vi "WaveformGen.vi"(7 "Name (\"\" to Use UUID)":string="WaveformGen") -> ()   [LabVIEW 2020, in "CSM-SimWaveform.lvlib"]
doc: "------------- lvcsm -------------\n[CSMStates]\nItem 0 = \"Event Structure\"\nItem 1 = \"Idle\"\nItem 2 = \"CSM Documentation\"\nItem 3 = \"VI Reference\"\nItem 4 = \"Error Handler\"\nItem 5 = \"Critical Error\"\nItem 6 = \"Target Timeout Error\"\nItem 7 = \"Target Error\"\nItem 8 = \"Async Response\"\nItem 9 = \"Response\"\nItem 10 = \"Async Message Posted\"\nItem 11 = \"Initialize Core Data\"\nItem 12 = \"Exit\"\nItem 13 = \"Data: Initialize\"\nItem 14 = \"Data: Cleanup\"\nItem 15 = \"Events: Register\"\nItem 16 = \"Events: Unregister\"\nItem 17 = \"UI: Initialize\"\nItem 18 = \"UI: Cursor Set\"\nItem 19 = \"UI: Front Panel State\"\nItem 20 = \"Macro: Initialize\"\nItem 21 = \"Macro: Exit\"\nItem 22 = \"API: Configure\"\nItem 23 = \"API: Start\"\nItem 24 = \"API: Stop\"\nItem 25 = \"Action: GenerateWaveforms\"\n\n[CSMStatus]\nItem 0 = \"Acquired Waveform@\"\nItem 1 = \"Error Occurred@Error Handler\""
uses:
  _support/WfGenConf--Cluster.ctl
  d2f34d03-87f3-4da2-90aa-e537ed74afc7.vi
  29d10371-2bcf-4fcf-9d9e-e563f382a514.vi
  <userlib>/_NEVSTOP/Communicable State Machine(CSM)/AdvanceAPI/CSM - Revert Arguments-Safe String.vi
  <userlib>/_NEVSTOP/Communicable State Machine(CSM)/_Shared/Trim Single-line Text.vi
  <userlib>/_NEVSTOP/Communicable State Machine(CSM)/AdvanceAPI/CSM - Make String Arguments Safe.vi
  <userlib>/_NEVSTOP/Communicable State Machine(CSM)/AdvanceAPI/CSM - Break Down Multiple States String.vi
  <userlib>/_NEVSTOP/Communicable State Machine(CSM)/AdvanceAPI/CSM - Compact Multiple States.vi
  <userlib>/_NEVSTOP/Communicable State Machine(CSM)/AdvanceAPI/CSM - Keywords.vi
  <userlib>/_NEVSTOP/Communicable State Machine(CSM)/AdvanceAPI/CSM - List Modules.vi
  <userlib>/_NEVSTOP/Communicable State Machine(CSM)/Utility/CSM Data Type String.vi
  <userlib>/_NEVSTOP/Communicable State Machine(CSM)/addons/MassData-Parameter/_support/FGV-MassData(lvlibp).vi
  <userlib>/_NEVSTOP/Communicable State Machine(CSM)/addons/API-String-Arugments-Support/_Support/Convert API String Arguments to Data(variant).vi
  CSM-SimWaveform.lvlib
  <userlib>/_NEVSTOP/Communicable State Machine(CSM)/Communicable State Machine.lvlib
panel:
  in  "System Stop Button":bool
  in  "System Start Button":bool
  out "Running?":bool
  in  "Generate Rate":u32(knob)=17 scale=1.0..50.0
  out "diff(ms)":u32
  in  "WaveformGen Settings":T1(array[cluster])=[{"sampling info"={"Fs"=1000.0, "#s"=1000.0}, "phase"=0.0, "amplitude"=1.0, "frequency"=10.0, "range"=1.0, "Type"=enum."Sine", "Waveform Name"="Waveform 0"}, {"sampling info"={"Fs"=1000.0, "#s"=1000.0}, "phase"=0.0, "amplitude"=1.0, "frequency"=10.0, "range"=1.0, "Type"=enum."Triangle", "Waveform Name"="Waveform 1"}, {"sampling info"={"Fs"=1000.0, "#s"=1000.0}, "phase"=0.0, "amplitude"=1.0, "frequency"=10.0, "range"=1.0, "Type"=enum."Sawtooth", "Waveform Name"="Waveform 2"}, {"sampling info"={"Fs"=1000.0, "#s"=1000.0}, "phase"=0.0, "amplitude"=1.0, "frequency"=10.0, "range"=1.0, "Type"=enum."Square", "Waveform Name"="Waveform 3"}]
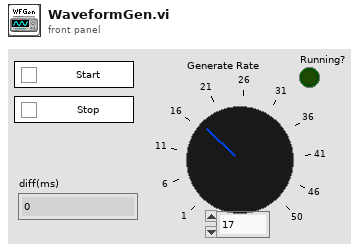
[diagram p1: front panel]
types:
  T1 = cluster{"sampling info":cluster{"Fs":dbl, "#s":dbl}, "phase":dbl, "amplitude":dbl, "frequency":dbl, "range":dbl, "Type":enum16{"Sine", "Triangle", "Sawtooth", "Square"}, "Waveform Name":string}[]
  T2 = enum32{"Invalid", "Standard", "Closed", "Hidden", "Minimized", "Maximized"}
  T3 = enum32{"invalid app kind", "Development System", "Run Time System", "Student Edition", "Embedded LabVIEW", "Evaluation", "Custom"}
  T4 = typedef "Communicable State Machine.lvlib/_CSM_Response Source Message.ctl" = cluster{"‘State":string, "’Arguments":string, "’Error":errorcluster}
  T5 = cluster{"Current VI Reference":refnum<vi>, "Close Panel on Exit?":bool}
  T6 = typedef "CSM-SimWaveform.lvlib/WfGenConf--Cluster.ctl" = cluster{"WaveformGen Settings":cluster{"sampling info":cluster{"Fs":dbl, "#s":dbl}, "phase":dbl, "amplitude":dbl, "frequency":dbl, "range":dbl, "Type":enum16{"Sine", "Triangle", "Sawtooth", "Square"}, "Waveform Name":string}[], "Generate Rate":dbl, "Gen?":bool}
  T7 = cluster{"Core":cluster{"Current VI Reference":refnum<vi>, "Close Panel on Exit?":bool}, "Configuration":T6}
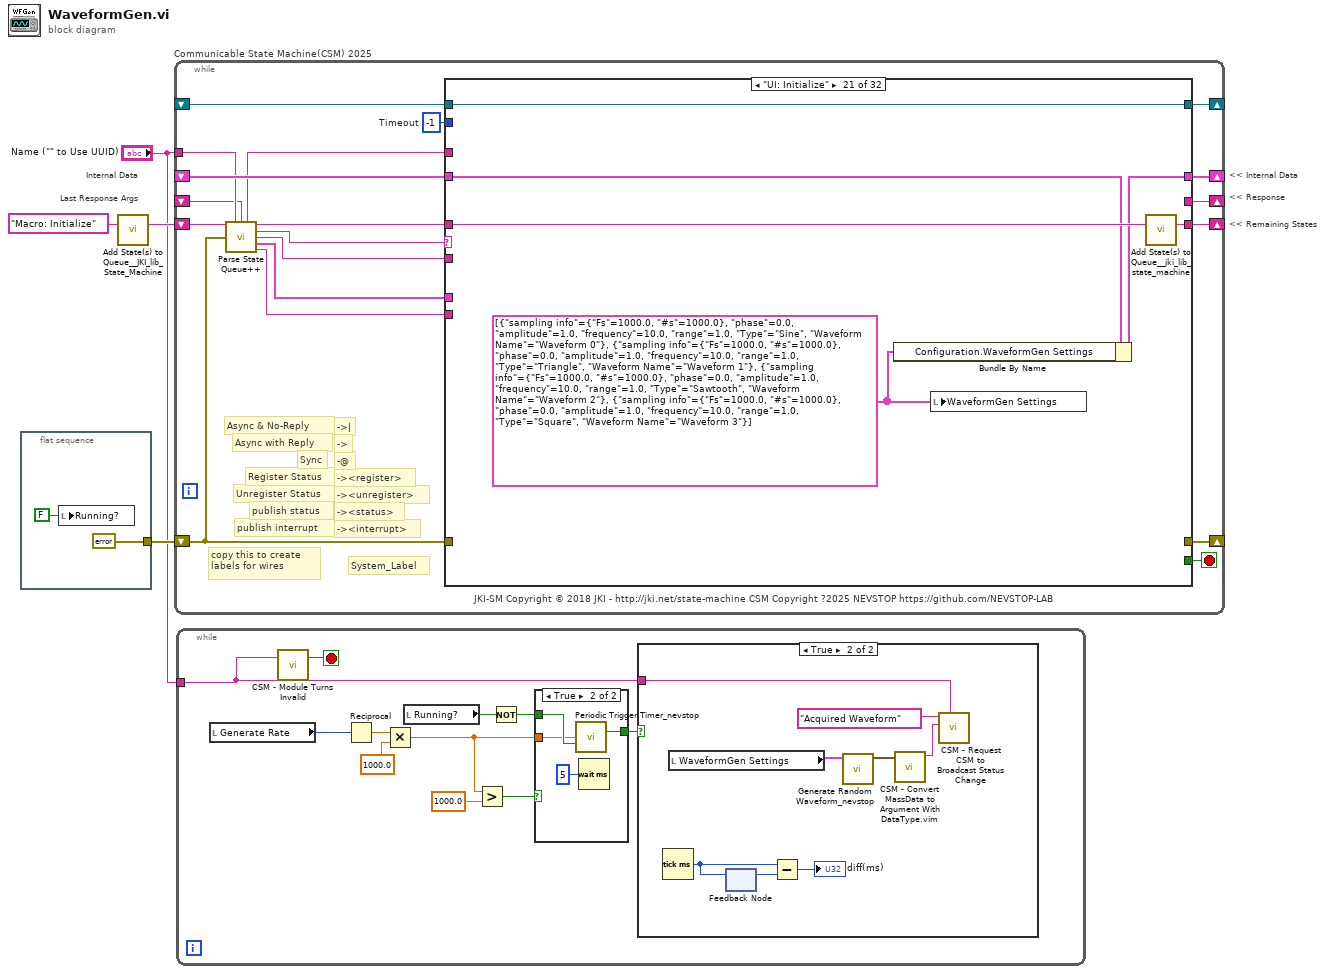
[diagram p0: block diagram]
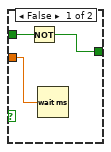
[diagram p2: hidden frame]
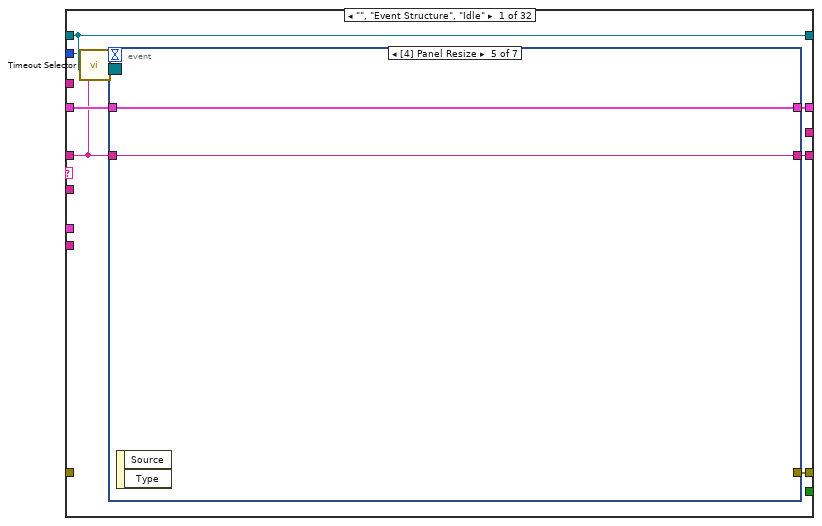
[diagram p4: hidden frame]
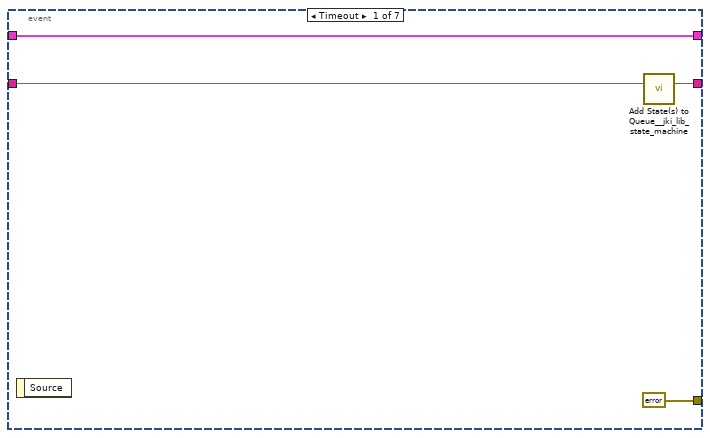
[diagram p5: hidden frame]
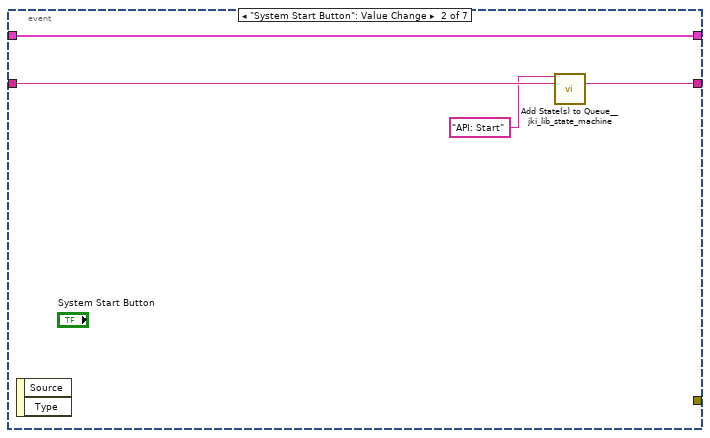
[diagram p6: hidden frame]
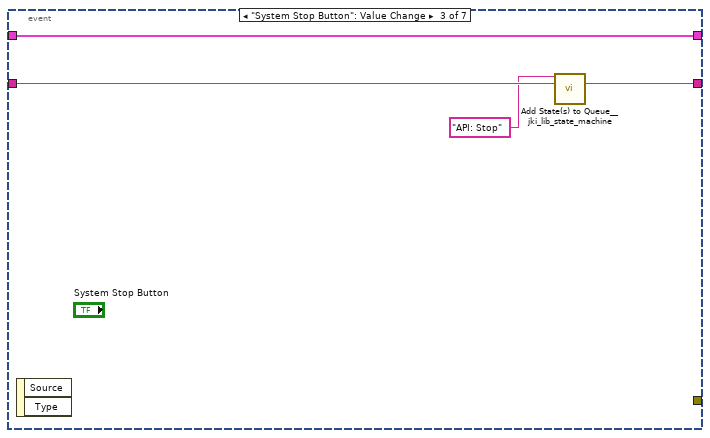
[diagram p7: hidden frame]
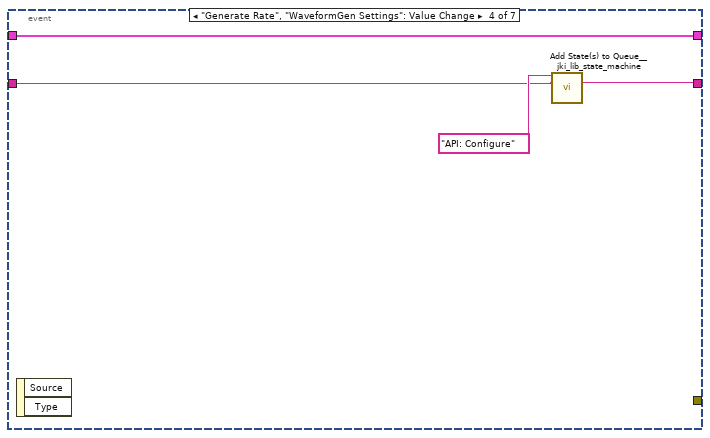
[diagram p8: hidden frame]
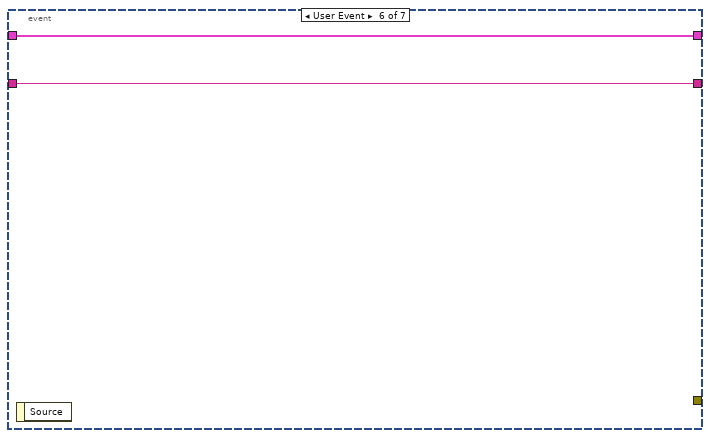
[diagram p9: hidden frame]
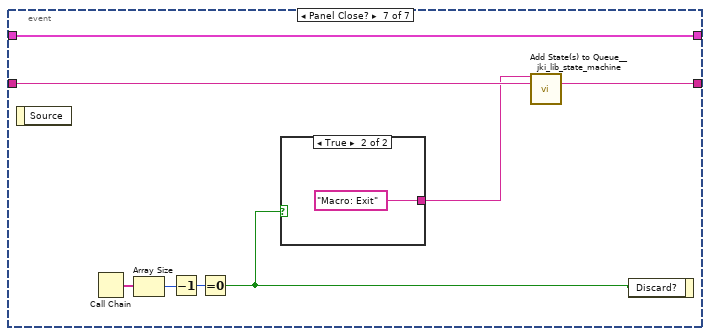
[diagram p10: hidden frame]
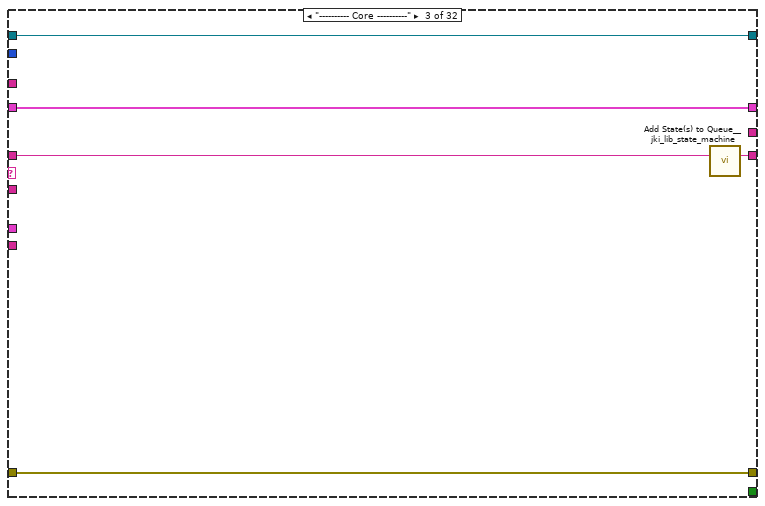
[diagram p13: hidden frame]
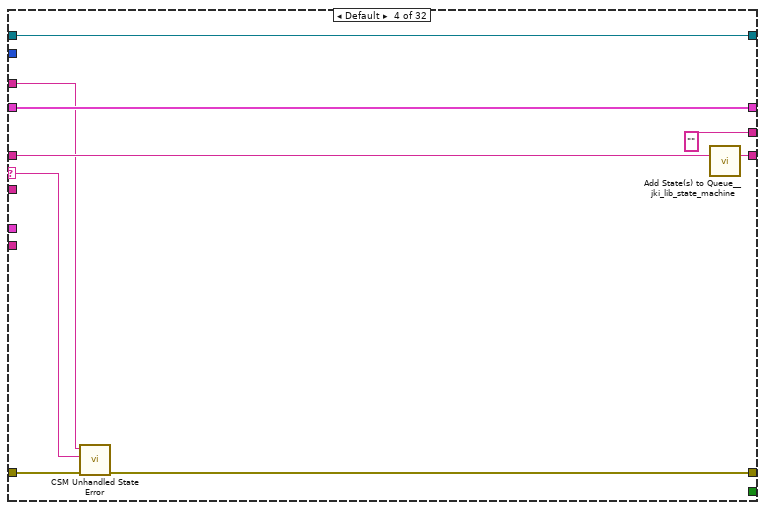
[diagram p14: hidden frame]
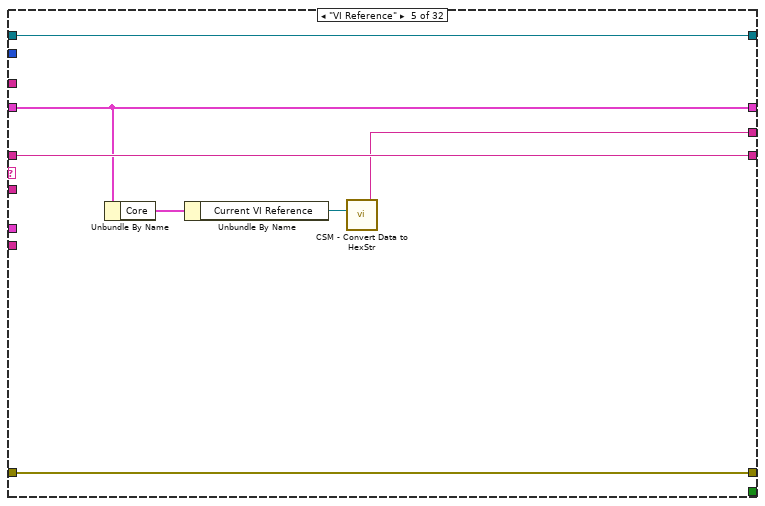
[diagram p15: hidden frame]
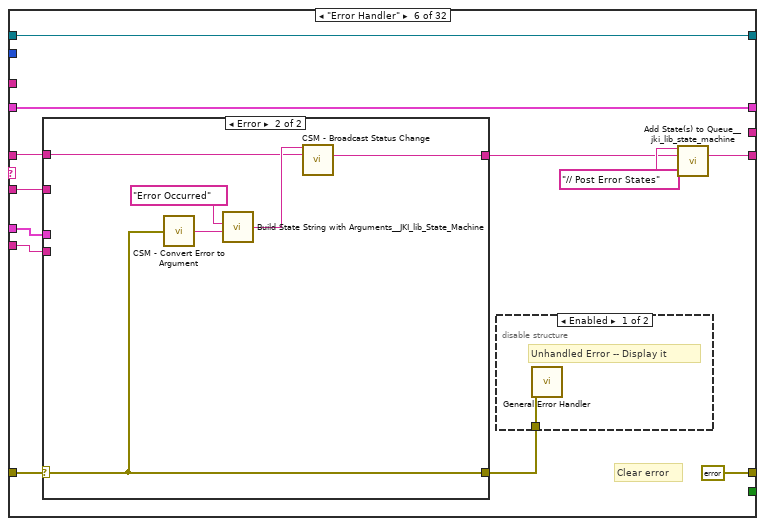
[diagram p16: hidden frame]
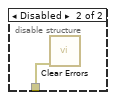
[diagram p17: hidden frame]
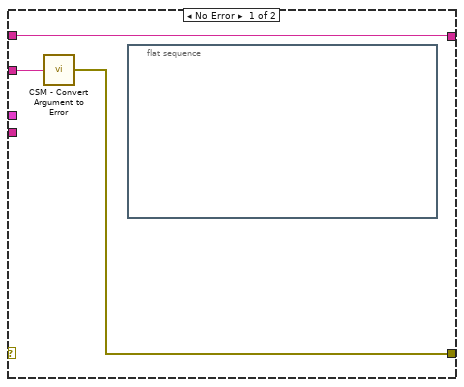
[diagram p18: hidden frame]
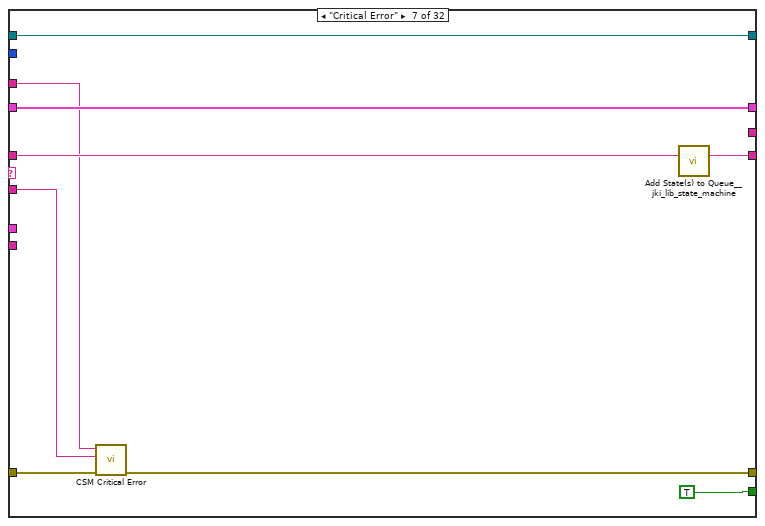
[diagram p19: hidden frame]
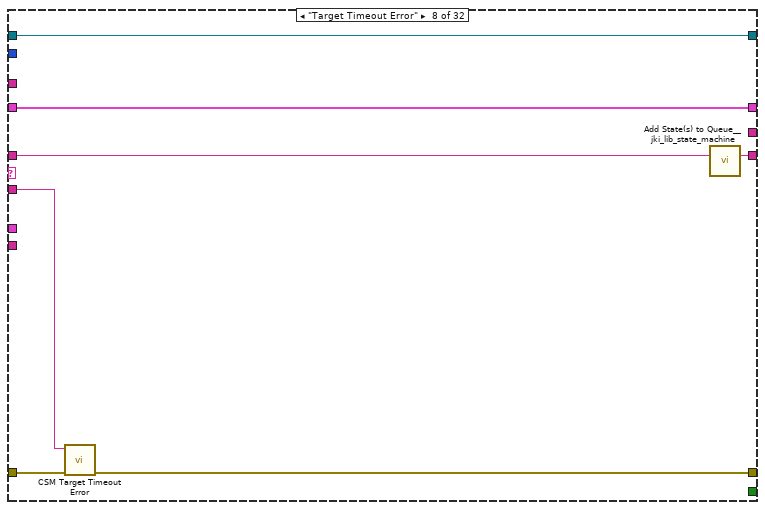
[diagram p20: hidden frame]
diagram:
  # "Last Response Args"
  # "Internal Data"
  # "<< Internal Data"
  # "<< Response"
  # "<< Remaining States"
  n1 = flat-sequence {
    tunnel: [errorcluster {"status"=FALSE, "code"=0, "source"=""} ("error out")] -> w4
    frame #0 {
      n2 = local write "Running?"(FALSE ("Running?")) -> ()
    }
  }
  n3 = call <vilib>:"Add State(s) to Queue__JKI_lib_State_Machine.vi"("State(s) in (\"\")"="Macro: Initialize" ("Init State(\"Macro: Initialize\")")) -> ("States Out"=w2:string)  [unwired: 14 in]
  n4 = while "Communicable State Machine(CSM) 2025" {
    shift-right: [w20] -> _
    shift-left: _ -> [w19]
    shift-right: [w23] -> _
    shift-left: w4 -> [w17]
    shift-right: [w22] -> _
    shift-left: w2 -> [w24]
    tunnel: "Name (\"\" to Use UUID)" -> [w13]
    shift-right: [w16] -> _
    shift-left: _ -> [w8]
    shift-right: [w15] -> _
    shift-left: _ -> [w14]
    stop <- w21 stop-if-true
    w18 = -1  # Timeout
    # "-><interrupt>"
    # "-><status>"
    # "-><unregister>"
    # "-><register>"
    # "-@"
    # "->"
    # "->|"
    # "publish interrupt"
    # "publish status"
    # "Unregister Status"
    # "Register Status"
    # "Sync"
    # "Async with Reply"
    # "Async & No-Reply"
    # "copy this to create labels for wires"
    # "System_Label"
    # "JKI-SM Copyright © 2018 JKI - http://jki.net/state-machine CSM Copyright ?2025 NEVSTOP https://github.com/NEVSTOP-LAB"
    n5 = call <userlib>:"Parse State Queue++.vi"("State Queue"=w24, "Name (\"\" to Use UUID)"=w13, "Response Arguments"=w8, "Previous Error"=w17) -> ("Name Used"=w9:string, "Remaining States"=w25:string, "Current State"=w12:string, "Arguments"=w7:string, "Additional Information"=w11:T4, "Source CSM"=w10:string)  [unwired: 6 in]
    n6 = case shown="\"UI: Initialize\"" w12 {
      selector: w12 -> [_ _ _ w73 _ _ _ _ _ _ _ _ _ _ _ _ _ _ _ _ _ _ _ _ _ _ _ _ _ _ _ _]
      tunnel: w25 -> [w26 w65 w70 w79 w85 w91 w117 w125 w132 w142 w151 w164 w169 w173 w179 w185 w189 w196 w200 w204 w210 w216 w227 w291 w296 w307 w310 w319 w323 w327 w331 w335]
      tunnel: w7 -> [_ _ _ _ _ w89 w113 w120 w128 w136 _ _ _ _ _ _ _ _ _ _ _ w212 w222 _ _ _ _ w312 _ _ _ _]
      tunnel: w19 -> [w32 w64 w67 w77 w84 w97 w118 w123 w130 w140 w150 w158 w167 w171 _ w181 w187 w195 w199 w202 w208 w214 w224 w289 w294 w305 w309 w314 w322 w326 w329 w332]
      tunnel: [w31 _ w68 w71 w86 errorcluster {"status"=FALSE, "code"=0, "source"=""} ("error out") w110 w119 w126 w139 _ _ _ _ _ w182 _ w190 w198 _ _ w213 w225 _ _ _ _ w311 _ _ _ _] -> w23
      tunnel: w17 -> [_ _ w68 w72 w86 w95 w111 w121 w127 _ _ _ _ _ _ _ _ _ _ _ _ _ _ _ _ _ _ _ _ _ _ _]
      tunnel: [w33 w65 w69 w78 w85 w93 w116 w124 w131 w143 w151 w163 w168 w172 w178 w184 w188 w196 w200 w203 w209 w215 w226 w290 w295 w306 w310 w319 w323 w327 w330 w334] -> w22
      tunnel: [_ _ _ _ _ _ TRUE _ _ _ _ _ TRUE _ _ _ _ _ _ _ _ _ _ _ _ _ _ _ _ _ _ _] -> w21
      tunnel: [w30 w64 w67 w77 w84 w97 w118 w123 w130 w141 w150 w162 w167 w171 w177 w181 w187 w195 w199 w202 w206 w214 w224 w289 w294 w305 w309 w313 w322 w326 w329 w332] -> w20
      tunnel: w18 -> [w28 _ _ _ _ _ _ _ _ _ _ _ _ _ _ _ _ _ _ _ _ _ _ _ _ _ _ _ _ _ _ _]
      tunnel: w10 -> [_ _ _ _ _ w88 _ _ _ w137 _ _ _ _ _ _ _ _ _ _ _ _ _ _ _ _ _ _ _ _ _ _]
      tunnel: w11 -> [_ _ _ _ _ w87 _ _ _ w138 _ _ _ _ _ _ _ _ _ _ _ _ _ _ _ _ _ _ _ _ _ _]
      tunnel: [_ _ _ "" w80 _ _ _ _ _ _ _ _ _ _ _ _ _ _ _ _ _ _ _ _ _ _ _ _ _ _ _] -> w16
      tunnel: [w29 w63 w66 w75 w83 w96 w114 w122 w129 w144 w149 w152 w165 w170 w175 w180 w186 w194 w197 w201 w207 w211 w221 w288 w292 w298 w308 w318 w321 w325 w328 w333] -> w15
      tunnel: w14 -> [w29 w63 w66 w75 w83 w96 w114 w122 w129 w144 w149 w152 w165 w170 w175 w180 w186 _ w197 w201 w207 w211 w221 w288 w292 w298 w308 w318 w321 w325 w328 w333]
      tunnel: w9 -> [_ _ _ w74 _ _ w112 _ _ _ _ _ _ _ _ _ _ w193 _ _ _ _ _ _ _ _ _ _ _ _ _ _]
      frame "", "Event Structure", "Idle" {
        n7 = call <userlib>:"Timeout Selector.vi"("Remaining States"=w26, "Timeout Expected"=w28) -> ("Timeout"=w27:i32)  [unwired: 5 in]
        n8 = event shown="[4] Panel Resize" {
          selector: w29 -> [_ _ _ _ _ _ _]
          dyn-events: _ -> [_ _ _ _ _ _ _]
          timeout: w27 -> [_ _ _ _ _ _ _]
          tunnel: w26 -> [w37 w39 w43 w47 w51 w52 w61]
          tunnel: [w36 w40 w44 w46 w51 w52 w60] -> w33
          tunnel: w32 -> [w35 w41 w45 w49 w50 w53 w59]
          tunnel: [errorcluster {"status"=FALSE, "code"=0, "source"=""} ("error out") _ _ _ _ _ _] -> w31
          tunnel: [w35 w41 w45 w49 w50 w53 w59] -> w30
          event Timeout {
            n9 = event-data() -> ()  [unwired: 1 in, 1 out]
            n10 = call <vilib>:"Add State(s) to Queue__jki_lib_state_machine.vi"("State(s) in (\"\")"=w37) -> ("States Out"=w36:string)  [unwired: 14 in]
          }
          event "System Start Button": Value Change {
            n11 = event-data() -> ()  [unwired: 1 in, 2 out]
            n12 = call <vilib>:"Add State(s) to Queue__jki_lib_state_machine.vi"("State(s) in Front (\"\")"="API: Start" ("State(s) in Front (\"\")"), "State(s) in (\"\")"=w39) -> ("States Out"=w40:string)  [unwired: 13 in]
          }
          event "System Stop Button": Value Change {
            n13 = event-data() -> ()  [unwired: 1 in, 2 out]
            n14 = call <vilib>:"Add State(s) to Queue__jki_lib_state_machine.vi"("State(s) in Front (\"\")"="API: Stop" ("State(s) in Front (\"\")"), "State(s) in (\"\")"=w43) -> ("States Out"=w44:string)  [unwired: 13 in]
          }
          event "Generate Rate", "WaveformGen Settings": Value Change {
            n15 = event-data() -> ()  [unwired: 1 in, 2 out]
            n16 = call <vilib>:"Add State(s) to Queue__jki_lib_state_machine.vi"("State(s) in Front (\"\")"="API: Configure" ("State(s) in Front (\"\")"), "State(s) in (\"\")"=w47) -> ("States Out"=w46:string)  [unwired: 13 in]
          }
          event Panel Resize {
            n17 = event-data() -> ()  [unwired: 1 in, 2 out]
          }
          event User Event {
            n18 = event-data() -> ()  [unwired: 1 in, 1 out]
          }
          event Panel Close? {
            n19 = event-data() -> ()  [unwired: 1 in, 1 out]
            n20 = Call Chain() -> (call chain=w58:string[])
            n21 = Array Size(array=w58) -> (size(s)=w57:i32)
            n22 = Decrement(x=w57) -> (x-1=w56:i32)
            n23 = Equal To 0?(x=w56) -> (x = 0?=w55:bool)
            n24 = case shown="True" w55 {
              tunnel: [_ "Macro: Exit"] -> w54
              frame False {
              }
              frame True {
              }
            }
            n25 = call <vilib>:"Add State(s) to Queue__jki_lib_state_machine.vi"("State(s) in Front (\"\")"=w54, "State(s) in (\"\")"=w61) -> ("States Out"=w60:string)  [unwired: 13 in]
            n26 = event-data("Discard?"=w55) -> ()  [unwired: 1 in, 1 out]
          }
        }
      }
      frame "CSM Documentation" {
      }
      frame "---------- Core ----------" {
        n27 = call <vilib>:"Add State(s) to Queue__jki_lib_state_machine.vi"("State(s) in (\"\")"=w70) -> ("States Out"=w69:string)  [unwired: 14 in]
      }
      frame Default {
        n28 = call <userlib>:"CSM Unhandled State Error.vi"("error in (no error)"=w72, "Undefined State"=w73, "CSM Name"=w74) -> ("error out"=w71:errorcluster)  [unwired: 8 in]
        n29 = call <vilib>:"Add State(s) to Queue__jki_lib_state_machine.vi"("State(s) in (\"\")"=w79) -> ("States Out"=w78:string)  [unwired: 14 in]
      }
      frame "VI Reference" {
        n30 = Unbundle By Name(w84) -> ("Core"=w82:T5)
        n31 = Unbundle By Name(w82) -> ("Current VI Reference"=w81:refnum<vi>)
        n32 = call <userlib>:"CSM - Convert Data to HexStr.vi"("Variant"=w81) -> ("HEX String (0-9,A-F)"=w80:string)  [unwired: 8 in]
      }
      frame "Error Handler" {
        # "Clear error"
        n33 = case shown="Error" w95 {
          selector: w95 -> [_ w104]
          tunnel: [w102 w106] -> w92
          tunnel: w91 -> [w102 w105]
          tunnel: [w101 w104] -> w90
          tunnel: w89 -> [w103 _]
          tunnel: w88 -> [_ _]
          tunnel: w87 -> [_ _]
          frame No Error {
            n34 = call <userlib>:"CSM - Convert Argument to Error.vi"("Argument"=w103) -> ("Error"=w101:errorcluster)  [unwired: 4 in]
            n35 = flat-sequence {
              frame #0 {
              }
            }
          }
          frame Error {
            n36 = call <userlib>:"CSM - Convert Error to Argument.vi"("Error"=w104) -> ("Argument"=w108:string)  [unwired: 4 in]
            n37 = call <vilib>:"Build State String with Arguments__JKI_lib_State_Machine.vi"("Arguments (\"\")"=w108, "State"="Error Occurred" ("Status with Arguments")) -> ("State with Arguments"=w107:string)  [unwired: 4 in]
            n38 = call <userlib>:"CSM - Broadcast Status Change.vi"("Status With Arguments"=w107, "State Queue"=w105) -> ("Remaining States"=w106:string)  [unwired: 13 in]
          }
        }
        n39 = disable-structure shown="Enabled" {
          disable-tunnel: w90 -> [w99 w100]
          frame Enabled {
            # "Unhandled Error -- Display it"
            n40 = call <vilib>:"General Error Handler.vi"("error in (no error)"=w99) -> ()  [unwired: 10 in, 5 out]
          }
          frame Disabled {
            n41 = call <vilib>:"Clear Errors.vi"("error in (no error)"=w100) -> ()  [unwired: 5 in, 2 out]
          }
        }
        n42 = call <vilib>:"Add State(s) to Queue__jki_lib_state_machine.vi"("State(s) in Front (\"\")"="// Post Error States", "State(s) in (\"\")"=w92) -> ("States Out"=w93:string)  [unwired: 13 in]
      }
      frame "Critical Error" {
        n43 = call <userlib>:"CSM Critical Error.vi"("error in (no error)"=w111, "Arugments (As Reason)"=w113, "CSM Name"=w112) -> ("error out"=w110:errorcluster)  [unwired: 8 in]
        n44 = call <vilib>:"Add State(s) to Queue__jki_lib_state_machine.vi"("State(s) in (\"\")"=w117) -> ("States Out"=w116:string)  [unwired: 14 in]
      }
      frame "Target Timeout Error" {
        n45 = call <userlib>:"CSM Target Timeout Error.vi"("error in (no error)"=w121, "Arguments (As CSM Name)"=w120) -> ("error out"=w119:errorcluster)  [unwired: 9 in]
        n46 = call <vilib>:"Add State(s) to Queue__jki_lib_state_machine.vi"("State(s) in (\"\")"=w125) -> ("States Out"=w124:string)  [unwired: 14 in]
      }
      frame "Target Error" {
        n47 = call <userlib>:"CSM Target Error.vi"("error in (no error)"=w127, "Arguments (As CSM Name)"=w128) -> ("error out"=w126:errorcluster)  [unwired: 9 in]
        n48 = call <vilib>:"Add State(s) to Queue__jki_lib_state_machine.vi"("State(s) in (\"\")"=w132) -> ("States Out"=w131:string)  [unwired: 14 in]
      }
      frame "Async Response", "Response" {
        n49 = Unbundle(w138) -> ("‘State"=w135:string, "’Arguments"=w134:string, "’Error"=w133:errorcluster)
        n50 = case shown="Default" w135 {
          tunnel: [w145] -> w143
          tunnel: w142 -> [w146]
          tunnel: [w148] -> w141
          tunnel: w140 -> [w148]
          tunnel: [w147] -> w139
          tunnel: w133 -> [w147]
          tunnel: w137 -> [_]
          tunnel: w136 -> [_]
          tunnel: w134 -> [_]
          frame Default {
            n51 = call <vilib>:"Add State(s) to Queue__jki_lib_state_machine.vi"("State(s) in (\"\")"=w146) -> ("States Out"=w145:string)  [unwired: 14 in]
          }
        }
      }
      frame "Async Message Posted" {
      }
      frame "Initialize Core Data" {
        # "originally closed?"
        # "exe?"
        # "If panel starts closed or is an EXE, then close it when we exit"
        n52 = property class="VI"() -> ("FP.State"=w155:T2)  [unwired: 2 in, 2 out]
        n53 = property class="App"() -> ("App.Kind"=w161:T3)  [unwired: 2 in, 2 out]
        n54 = control-ref of="Current VI Reference"() -> (w156:refnum<vi>)
        n55 = Equal?(x=w155, y=T2."Closed" ("Front Panel Window:State")) -> (x = y?=w153:bool)
        n56 = Equal?(x=w161, y=T3."Run Time System" ("Application:Kind")) -> (x = y?=w159:bool)
        n57 = Or(x=w153, y=w159) -> (x .or. y?=w157:bool)
        n58 = Bundle By Name(cluster=w158, "Core.Current VI Reference"=w156, "Core.Close Panel on Exit?"=w157) -> (w162:T7)
        n59 = call <vilib>:"Add State(s) to Queue__jki_lib_state_machine.vi"("State(s) in (\"\")"=w164) -> ("States Out"=w163:string)  [unwired: 14 in]
      }
      frame "Exit" {
        n60 = call <vilib>:"Add State(s) to Queue__jki_lib_state_machine.vi"("State(s) in (\"\")"=w169) -> ("States Out"=w168:string)  [unwired: 14 in]
      }
      frame "---------- Data ----------" {
        n61 = call <vilib>:"Add State(s) to Queue__jki_lib_state_machine.vi"("State(s) in (\"\")"=w173) -> ("States Out"=w172:string)  [unwired: 14 in]
      }
      frame "Data: Initialize" {
        w174 = T6 {"WaveformGen Settings"=[], "Generate Rate"=10.0, "Gen?"=FALSE}  # Configuration
        w176 = T5 {"Current VI Reference"=refnum, "Close Panel on Exit?"=FALSE}  # Core
        n62 = Bundle("Core"=w176, "Configuration"=w174) -> (w177:T7)  [unwired: 1 in]
        n63 = call <vilib>:"Add State(s) to Queue__jki_lib_state_machine.vi"("State(s) in (\"\")"=w179) -> ("States Out"=w178:string)  [unwired: 14 in]
      }
      frame "Data: Cleanup" {
        n64 = Unbundle By Name(w181) -> ("Core.Current VI Reference"=w183:refnum<vi>)
        n65 = Close Reference(reference=w183) -> (error out=w182:errorcluster)  [unwired: 1 in]
        n66 = call <vilib>:"Add State(s) to Queue__jki_lib_state_machine.vi"("State(s) in (\"\")"=w185) -> ("States Out"=w184:string)  [unwired: 14 in]
      }
      frame "---------- Events ----------" {
        n67 = call <vilib>:"Add State(s) to Queue__jki_lib_state_machine.vi"("State(s) in (\"\")"=w189) -> ("States Out"=w188:string)  [unwired: 14 in]
      }
      frame "Events: Register" {
        n68 = call <userlib>:"CSM - Get New State Notifier Event.vi"("Name (\"\" to Use UUID)"=w193) -> ("error out"=w191:errorcluster, "New State Notifier Event"=w192:refnum<user-event>)  [unwired: 9 in]
        n69 = register-events(error in=w191, w192) -> (reference out=w194:refnum<event-registration>, error out=w190:errorcluster)  [unwired: 1 in]
      }
      frame "Events: Unregister" {
        n70 = Unregister For Events(event registration refnum=w197) -> (error out=w198:errorcluster)  [unwired: 1 in]
      }
      frame "---------- UI ----------" {
        n71 = call <vilib>:"Add State(s) to Queue__jki_lib_state_machine.vi"("State(s) in (\"\")"=w204) -> ("States Out"=w203:string)  [unwired: 14 in]
      }
      frame "UI: Initialize" {
        w205 = T1 [{"sampling info"={"Fs"=1000.0, "#s"=1000.0}, "phase"=0.0, "amplitude"=1.0, "frequency"=10.0, "range"=1.0, "Type"=enum."Sine", "Waveform Name"="Waveform 0"}, {"sampling info"={"Fs"=1000.0, "#s"=1000.0}, "phase"=0.0, "amplitude"=1.0, "frequency"=10.0, "range"=1.0, "Type"=enum."Triangle", "Waveform Name"="Waveform 1"}, {"sampling info"={"Fs"=1000.0, "#s"=1000.0}, "phase"=0.0, "amplitude"=1.0, "frequency"=10.0, "range"=1.0, "Type"=enum."Sawtooth", "Waveform Name"="Waveform 2"}, {"sampling info"={"Fs"=1000.0, "#s"=1000.0}, "phase"=0.0, "amplitude"=1.0, "frequency"=10.0, "range"=1.0, "Type"=enum."Square", "Waveform Name"="Waveform 3"}] ("Settings")
        n72 = Bundle By Name(cluster=w208, "Configuration.WaveformGen Settings"=w205) -> (w206:T7)
        n73 = local write "WaveformGen Settings"(w205) -> ()
        n74 = call <vilib>:"Add State(s) to Queue__jki_lib_state_machine.vi"("State(s) in (\"\")"=w210) -> ("States Out"=w209:string)  [unwired: 14 in]
      }
      frame "UI: Cursor Set" {
        # "Argument"
        n75 = disable-structure shown="TARGET_TYPE!=Windows" {
          disable-tunnel: [w218 _] -> w213
          disable-tunnel: w212 -> [w217 _]
          frame condition #0 (active) {
            n76 = case shown="\"Idle\", Default" w217 {
              tunnel: [w219 w220] -> w218
              frame "Idle", Default {
                n77 = call <vilib>:"Unset Busy.vi"() -> ("error out"=w219:errorcluster)  [unwired: 11 in]
              }
              frame "Busy" {
                n78 = call <vilib>:"Set Busy.vi"() -> ("error out"=w220:errorcluster)  [unwired: 10 in, 1 out]
              }
            }
          }
          frame condition #1 {
          }
        }
        n79 = call <vilib>:"Add State(s) to Queue__jki_lib_state_machine.vi"("State(s) in (\"\")"=w216) -> ("States Out"=w215:string)  [unwired: 14 in]
      }
      frame "UI: Front Panel State" {
        # "Argument"
        n80 = Unbundle By Name(w224) -> ("Core.Current VI Reference"=w223:refnum<vi>)
        n81 = case shown="\"Minimize\", \"Minimized\"" w222 {
          tunnel: [w234 w247 w258 w270 w282] -> w225
          tunnel: w223 -> [w233 w245 w257 w269 w281]
          frame "Open", "Standard", Default {
            w228 = T2."Standard" ("State")
            n82 = property class="VI"(reference=w233) -> (reference out=w231:refnum<vi>, error out=w232:errorcluster, "FP.State"=w230:T2)  [unwired: 1 in]
            n83 = Not Equal?(x=w230, y=w228) -> (x != y?=w229:bool)
            n84 = case shown="True" w229 {
              tunnel: [w238 w240] -> w234
              tunnel: w232 -> [w237 w240]
              tunnel: w231 -> [w236 _]
              tunnel: w228 -> [w235 _]
              frame True {
                n85 = invoke class="VI" method="FP.Open"(reference=w236, error in=w237, "Activate"=TRUE, "State"=w235) -> (error out=w238:errorcluster)  [unwired: 1 in, 4 out]
              }
              frame False {
              }
            }
          }
          frame "Close", "Closed" {
            n86 = property class="VI"(reference=w245) -> (reference out=w244:refnum<vi>, error out=w246:errorcluster, "FP.State"=w242:T2)  [unwired: 1 in]
            n87 = Not Equal?(x=w242, y=T2."Closed" ("Front Panel Window:State")) -> (x != y?=w241:bool)
            n88 = case shown="True" w241 {
              tunnel: [w248 w251] -> w247
              tunnel: w246 -> [w248 w250]
              tunnel: w244 -> [_ w249]
              frame False {
              }
              frame True {
                n89 = invoke class="VI" method="FP.Close"(reference=w249, error in=w250) -> (error out=w251:errorcluster)  [unwired: 1 in, 2 out]
              }
            }
          }
          frame "Hidden", "Hide" {
            w252 = T2."Hidden" ("State")
            n90 = property class="VI"(reference=w257) -> (reference out=w255:refnum<vi>, error out=w256:errorcluster, "FP.State"=w254:T2)  [unwired: 1 in]
            n91 = Not Equal?(x=w254, y=w252) -> (x != y?=w253:bool)
            n92 = case shown="True" w253 {
              tunnel: [w262 w263] -> w258
              tunnel: w256 -> [w261 w263]
              tunnel: w255 -> [w260 _]
              tunnel: w252 -> [w259 _]
              frame True {
                n93 = invoke class="VI" method="FP.Open"(reference=w260, error in=w261, "State"=w259) -> (error out=w262:errorcluster)  [unwired: 2 in, 4 out]
              }
              frame False {
              }
            }
          }
          frame "Minimize", "Minimized" {
            w264 = T2."Minimized" ("State")
            n94 = property class="VI"(reference=w269) -> (reference out=w267:refnum<vi>, error out=w268:errorcluster, "FP.State"=w266:T2)  [unwired: 1 in]
            n95 = Not Equal?(x=w266, y=w264) -> (x != y?=w265:bool)
            n96 = case shown="False" w265 {
              tunnel: [w274 w275] -> w270
              tunnel: w268 -> [w273 w275]
              tunnel: w267 -> [w272 _]
              tunnel: w264 -> [w271 _]
              frame True {
                n97 = invoke class="VI" method="FP.Open"(reference=w272, error in=w273, "State"=w271) -> (error out=w274:errorcluster)  [unwired: 2 in, 4 out]
              }
              frame False {
              }
            }
          }
          frame "Maximize", "Maximized" {
            w276 = T2."Maximized" ("State")
            n98 = property class="VI"(reference=w281) -> (reference out=w279:refnum<vi>, error out=w280:errorcluster, "FP.State"=w278:T2)  [unwired: 1 in]
            n99 = Not Equal?(x=w278, y=w276) -> (x != y?=w277:bool)
            n100 = case shown="True" w277 {
              tunnel: [w286 w287] -> w282
              tunnel: w280 -> [w285 w287]
              tunnel: w279 -> [w284 _]
              tunnel: w276 -> [w283 _]
              frame True {
                n101 = invoke class="VI" method="FP.Open"(reference=w284, error in=w285, "State"=w283) -> (error out=w286:errorcluster)  [unwired: 2 in, 4 out]
              }
              frame False {
              }
            }
          }
        }
        n102 = call <vilib>:"Add State(s) to Queue__jki_lib_state_machine.vi"("State(s) in (\"\")"=w227) -> ("States Out"=w226:string)  [unwired: 14 in]
      }
      frame "---------- Macro ----------" {
        n103 = call <vilib>:"Add State(s) to Queue__jki_lib_state_machine.vi"("State(s) in (\"\")"=w291) -> ("States Out"=w290:string)  [unwired: 14 in]
      }
      frame "Macro: Initialize" {
        w293 = "Data: Initialize\nInitialize Core Data\nEvents: Register\nUI: Initialize\n//UI: Front Panel State >> Open"  # Data: Initialize Initialize Core Data Events: Register UI: Initialize //UI: Front Panel State >> Open
        n104 = call <vilib>:"Add State(s) to Queue__jki_lib_state_machine.vi"("State(s) in Front (\"\")"=w293, "State(s) in (\"\")"=w296) -> ("States Out"=w295:string)  [unwired: 13 in]
      }
      frame "Macro: Exit" {
        w303 = "UI: Front Panel State >> Close"  # UI: Front Panel State >> Close
        n105 = Unbundle By Name(w305) -> ("Core.Close Panel on Exit?"=w304:bool)
        n106 = Select(t=w303, s=w304, f="") -> (s? t:f=w301:string)
        n107 = call <vilib>:"Add State(s) to Queue__jki_lib_state_machine.vi"("State(s) in Front (\"\")"="//Exit Sub-Modules ", "State(s) in (\"\")"=w301, "State(s) at Back (\"\")"="Data: Cleanup\nEvents: Unregister\nExit") -> ("States Out"=w299:string)  [unwired: 12 in]
        n108 = call <vilib>:"Add State(s) to Queue__jki_lib_state_machine.vi"("State(s) in Front (\"\")"=w299, "State(s) in (\"\")"=w307) -> ("States Out"=w306:string)  [unwired: 13 in]
      }
      frame "---------- API ----------" {
      }
      frame "API: Configure" {
        n109 = Bundle By Name(cluster=w314, "Configuration.WaveformGen Settings"="WaveformGen Settings", "Configuration.Generate Rate"="Generate Rate") -> (w317:T7)
        n110 = call "Convert API String Arguments to Data.vim"("Reference Type"=w317, "API String"=w312) -> ("error out"=w311:errorcluster, "Data"=w313:T7)  [unwired: 6 in]
      }
      frame "API: Start" {
        "Running?" <- TRUE ("Running?")
      }
      frame "API: Stop" {
        n111 = local write "Running?"(FALSE ("Configuration.Gen?")) -> ()
      }
      frame "---------- Action ----------" {
        n112 = call <vilib>:"Add State(s) to Queue__jki_lib_state_machine.vi"("State(s) in (\"\")"=w331) -> ("States Out"=w330:string)  [unwired: 14 in]
      }
      frame "Action: GenerateWaveforms" {
        n113 = call <vilib>:"Add State(s) to Queue__jki_lib_state_machine.vi"("State(s) in (\"\")"=w335) -> ("States Out"=w334:string)  [unwired: 14 in]
      }
    }
  }
  n114 = while {
    tunnel: "Name (\"\" to Use UUID)" -> [w340]
    stop <- w341 stop-if-true
    n115 = local read "Generate Rate"() -> (w342:u32)
    n116 = call <userlib>:"CSM - Module Turns Invalid.vi"("CSM Name"=w340) -> ("Turn Invalid (Exit)?"=w341:bool)  [unwired: 2 in]
    n117 = Reciprocal(x=w342) -> (1/x=w344:dbl)
    n118 = Multiply(x=w344, y=1000.0) -> (x*y=w338:dbl)
    n119 = local read "Running?"() -> (w343:bool)
    n120 = Greater?(x=w338, y=1000.0) -> (0:w336:bool)
    n121 = Not(x=w343) -> (.not. x?=w345:bool)
    n122 = case shown="True" w336 {
      tunnel: w345 -> [w348 w352]
      tunnel: [w347 w351] -> w339
      tunnel: w338 -> [w349 w350]
      frame False {
        n123 = Not(x=w348) -> (.not. x?=w347:bool)
        n124 = Wait (ms)(milliseconds to wait=w349) -> ()  [unwired: 1 out]
      }
      frame True {
        n125 = call <userlib>:"Periodic Trigger Timer_nevstop.vi"("time (ms)"=w350, "reset"=w352) -> ("Triggered"=w351:bool)  [unwired: 11 in, 2 out]
        n126 = Wait (ms)(milliseconds to wait=u32 5) -> ()  [unwired: 1 out]
      }
    }
    n127 = case shown="True" w339 {
      tunnel: w340 -> [_ w361]
      frame False {
      }
      frame True {
        n128 = Tick Count (ms)() -> (millisecond timer value=w357:u32)
        n129 = local read "WaveformGen Settings"() -> (w354:T1)
        n130 = feedback #1() -> (w358:u32)  [unwired: 1 in]
        n131 = feedback-in #1(w357) -> ()
        n132 = Subtract(x=w357, y=w358) -> (x-y=→"diff(ms)":u32)
        n133 = call <userlib>:"Generate Random Waveform_nevstop.vi"("WaveformGen Settings"=w354) -> ("Waveforms"=w356:waveform(dbl)[])  [unwired: 9 in, 1 out]
        n134 = call "CSM - Convert MassData to Argument With DataType.vim"("Data"=w356) -> ("MassData Argument"=w355:string)  [unwired: 7 in, 1 out]
        n135 = call <userlib>:"CSM - Request CSM to Broadcast Status Change.vi"("Module Name"=w361, "Arguments (\"\")"=w355, "Status"="Acquired Waveform" ("TRUE(Empty)")) -> ()  [unwired: 8 in, 1 out]
      }
    }
  }
